vi "Test VI.vi"() -> ()   [LabVIEW 2022 SP3]
panel:
  in  "Input":dbl
  out "Numeric":dbl
  in  "error in (no error)":errorcluster
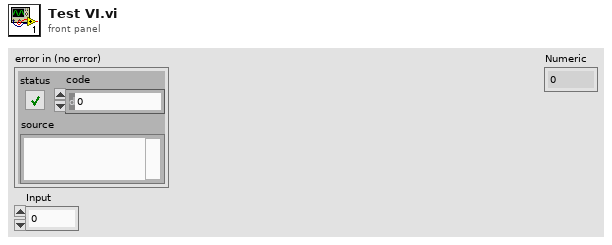
[diagram p1: front panel]
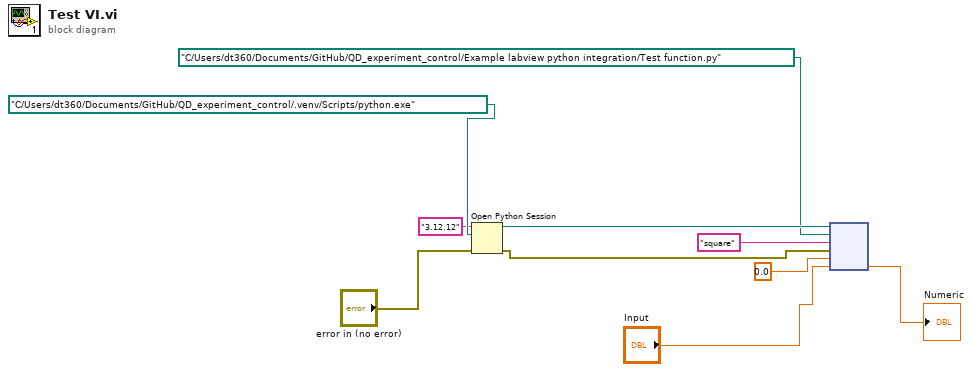
[diagram p0: block diagram]
diagram:
  n1 = Open Python Session(python version="3.12.12" ("Python version"), python path=path "C:/Users/dt360/Documents/GitHub/QD_experiment_control/.venv/Scripts/python.exe" ("Python path"), 3:"error in (no error)") -> (session out=w8:refnum<k35>, error out=w5:errorcluster)
  n2 = node(w8, path "C:/Users/dt360/Documents/GitHub/QD_experiment_control/Example labview python integration/Test function.py" ("module path"), "square" ("function name"), w5, 0.0, "Input") -> (→"Numeric":dbl)  [unwired: 1 in, 4 out]
